vi "4461 - AO Write Data.vi"(8 "error in":errorcluster, 10 "AO Array":waveform(dbl)[](array[waveform]), 11 "AO Task":refnum<k21>[](array[refnum])) -> (0 "error out":errorcluster)   [LabVIEW 2013]
uses:
  <vilib>/DAQmx/write.llb/DAQmx Write (Analog 1D Wfm NChan NSamp).vi
  <vilib>/DAQmx/miscellaneous.llb/DAQmx Fill In Error Info.vi
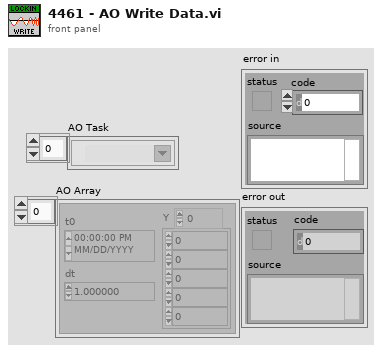
[diagram p1: front panel]
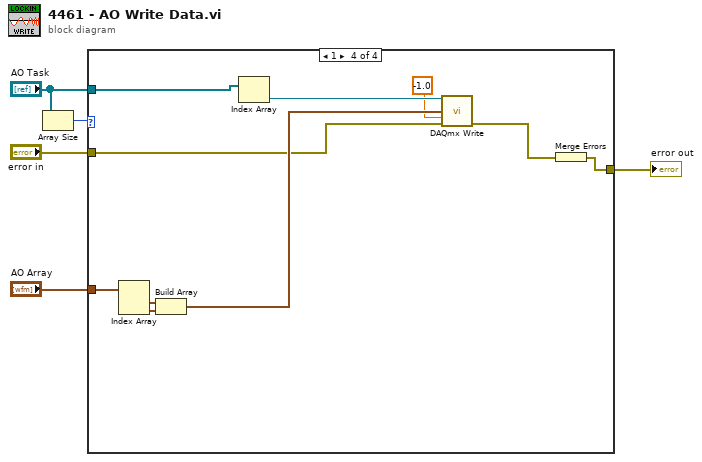
[diagram p0: block diagram]
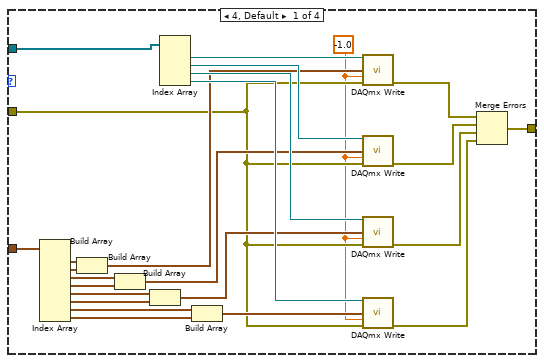
[diagram p2: hidden frame]
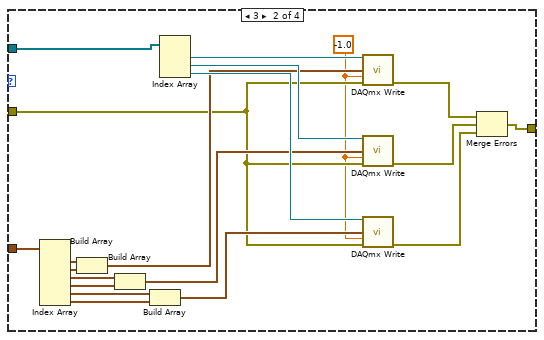
[diagram p3: hidden frame]
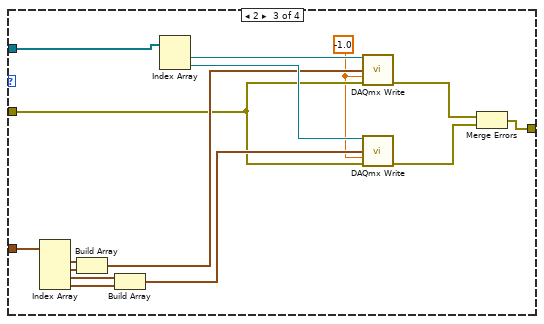
[diagram p4: hidden frame]
diagram:
  n1 = Array Size(array="AO Task") -> (size(s)=w1:i32)
  n2 = case shown="1" w1 {
    tunnel: "AO Array" -> [w29 w50 w65 w75]
    tunnel: "AO Task" -> [w28 w49 w64 w74]
    tunnel: "error in" -> [w12 w36 w55 w69]
    tunnel: [w7 w32 w52 w67] -> w3
    frame 4, Default {
      w6 = -1.0 ("timeout")
      n3 = Index Array(array=w29) -> (element #1=w23:waveform(dbl), element #2=w22:waveform(dbl), element #3=w21:waveform(dbl), element #4=w20:waveform(dbl), element #5=w19:waveform(dbl), element #6=w18:waveform(dbl), element #7=w17:waveform(dbl), element #8=w16:waveform(dbl))  [unwired: 8 in]
      n4 = Build Array(w23, w22) -> (w15:waveform(dbl)[])
      n5 = Build Array(w21, w20) -> (w14:waveform(dbl)[])
      n6 = Build Array(w19, w18) -> (w13:waveform(dbl)[])
      n7 = Index Array(array=w28) -> (element #1=w27:refnum<k21>, element #2=w26:refnum<k21>, element #3=w25:refnum<k21>, element #4=w24:refnum<k21>)  [unwired: 4 in]
      n8 = Build Array(w17, w16) -> (w30:waveform(dbl)[])
      n9 = call-poly <vilib>:"DAQmx Write.vi"("task/channels in"=w27, "data"=w15, "timeout"=w6, "error in"=w12) -> ("error out"=w8:errorcluster)  [unwired: 9 in, 2 out]
      n10 = call-poly <vilib>:"DAQmx Write.vi"("task/channels in"=w26, "data"=w14, "timeout"=w6, "error in"=w12) -> ("error out"=w11:errorcluster)  [unwired: 9 in, 2 out]
      n11 = call-poly <vilib>:"DAQmx Write.vi"("task/channels in"=w25, "data"=w13, "timeout"=w6, "error in"=w12) -> ("error out"=w10:errorcluster)  [unwired: 9 in, 2 out]
      n12 = call-poly <vilib>:"DAQmx Write.vi"("task/channels in"=w24, "data"=w30, "timeout"=w6, "error in"=w12) -> ("error out"=w9:errorcluster)  [unwired: 9 in, 2 out]
      n13 = Merge Errors(w8, w11, w10, w9) -> (w7:errorcluster)
    }
    frame 3 {
      w31 = -1.0 ("timeout")
      n14 = Index Array(array=w50) -> (element #1=w45:waveform(dbl), element #2=w44:waveform(dbl), element #3=w43:waveform(dbl), element #4=w42:waveform(dbl), element #5=w41:waveform(dbl), element #6=w40:waveform(dbl))  [unwired: 6 in]
      n15 = Build Array(w45, w44) -> (w39:waveform(dbl)[])
      n16 = Build Array(w43, w42) -> (w38:waveform(dbl)[])
      n17 = Build Array(w41, w40) -> (w37:waveform(dbl)[])
      n18 = Index Array(array=w49) -> (element #1=w48:refnum<k21>, element #2=w47:refnum<k21>, element #3=w46:refnum<k21>)  [unwired: 3 in]
      n19 = call-poly <vilib>:"DAQmx Write.vi"("task/channels in"=w48, "data"=w39, "timeout"=w31, "error in"=w36) -> ("error out"=w33:errorcluster)  [unwired: 9 in, 2 out]
      n20 = call-poly <vilib>:"DAQmx Write.vi"("task/channels in"=w47, "data"=w38, "timeout"=w31, "error in"=w36) -> ("error out"=w35:errorcluster)  [unwired: 9 in, 2 out]
      n21 = call-poly <vilib>:"DAQmx Write.vi"("task/channels in"=w46, "data"=w37, "timeout"=w31, "error in"=w36) -> ("error out"=w34:errorcluster)  [unwired: 9 in, 2 out]
      n22 = Merge Errors(w33, w35, w34) -> (w32:errorcluster)
    }
    frame 2 {
      w51 = -1.0 ("timeout")
      n23 = Index Array(array=w65) -> (element #1=w61:waveform(dbl), element #2=w60:waveform(dbl), element #3=w59:waveform(dbl), element #4=w58:waveform(dbl))  [unwired: 4 in]
      n24 = Build Array(w61, w60) -> (w57:waveform(dbl)[])
      n25 = Build Array(w59, w58) -> (w56:waveform(dbl)[])
      n26 = Index Array(array=w64) -> (element #1=w63:refnum<k21>, element #2=w62:refnum<k21>)  [unwired: 2 in]
      n27 = call-poly <vilib>:"DAQmx Write.vi"("task/channels in"=w63, "data"=w57, "timeout"=w51, "error in"=w55) -> ("error out"=w53:errorcluster)  [unwired: 9 in, 2 out]
      n28 = call-poly <vilib>:"DAQmx Write.vi"("task/channels in"=w62, "data"=w56, "timeout"=w51, "error in"=w55) -> ("error out"=w54:errorcluster)  [unwired: 9 in, 2 out]
      n29 = Merge Errors(w53, w54) -> (w52:errorcluster)
    }
    frame 1 {
      n30 = Index Array(array=w75) -> (element #1=w72:waveform(dbl), element #2=w71:waveform(dbl))  [unwired: 2 in]
      n31 = Build Array(w72, w71) -> (w70:waveform(dbl)[])
      n32 = Index Array(array=w74) -> (element=w73:refnum<k21>)  [unwired: 1 in]
      n33 = call-poly <vilib>:"DAQmx Write.vi"("task/channels in"=w73, "data"=w70, "timeout"=-1.0, "error in"=w69) -> ("error out"=w68:errorcluster)  [unwired: 9 in, 2 out]
      n34 = Merge Errors(w68) -> (w67:errorcluster)
    }
  }
  "error out" <- w3
